vi "Destroy.vi"(0 "reference in":refnum<class "LcPictureBox.lvclass">, 5 "Error In":errorcluster) -> (14 "reference out":refnum<class "LcPictureBox.lvclass">, 19 "Error Out":errorcluster)   [LabVIEW 2020, in "LcPictureBox.lvclass"]
uses:
  LcPictureBox.lvclass
  System.Drawing
  System.Windows.Forms
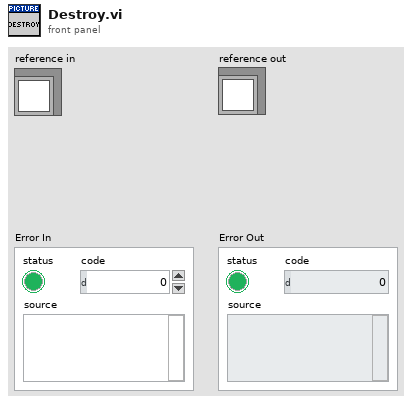
[diagram p1: front panel]
types:
  T1 = typedef "LcPictureBox.lvclass/ObjectAttributes.ctl" = cluster{"PictureBox":refnum<k24>, "ImageSize":cluster{"Width":i32, "Height":i32}, "PenMemory":map{cluster{"Alpha(100%)":dbl, "Color(Black)":u32, "Pen(Width=1, Solid)":T2}, refnum<k24>}, "GraphicsRef":refnum<k24>, "BrushMemory":map{cluster{"Alpha(100%)":dbl, "Color(Black)":u32}, refnum<k24>}, "Images":refnum<k24>[], "ImageIndex":i32, "BgColor(None)":u32, "LoadedImages":map{string, cluster{"ImageOut":refnum<k24>, "ImageSize":cluster{"Width":i32, "Height":i32}}}, "ColorsMemory":map{cluster{"Alpha(100%)":dbl, "Color(Black)":u32}, refnum<k24>}, "CacheSize":i32, "PictureBoxActiveXReference":refnum<vi>, "Scale":dbl, "Offset":cluster{"x":sgl, "y":sgl}, "zoom_center":cluster{"X":i32, "Y":i32}, "ImagesCreated":refnum<k24>[], "CustomCursorImages":map{u16, refnum<k24>}}
  T2 = typedef "LcPictureBox.lvclass/Pen.ctl" = cluster{"Width":u16, "Style":enum32{"Solid", "Dash", "Dot", "DashDot", "DashDotDot"}}
  T3 = map{cluster{"Alpha(100%)":dbl, "Color(Black)":u32}, refnum<k24>}
  T4 = map{cluster{"Alpha(100%)":dbl, "Color(Black)":u32, "Pen(Width=1, Solid)":T2}, refnum<k24>}
  T5 = map{string, cluster{"ImageOut":refnum<k24>, "ImageSize":cluster{"Width":i32, "Height":i32}}}
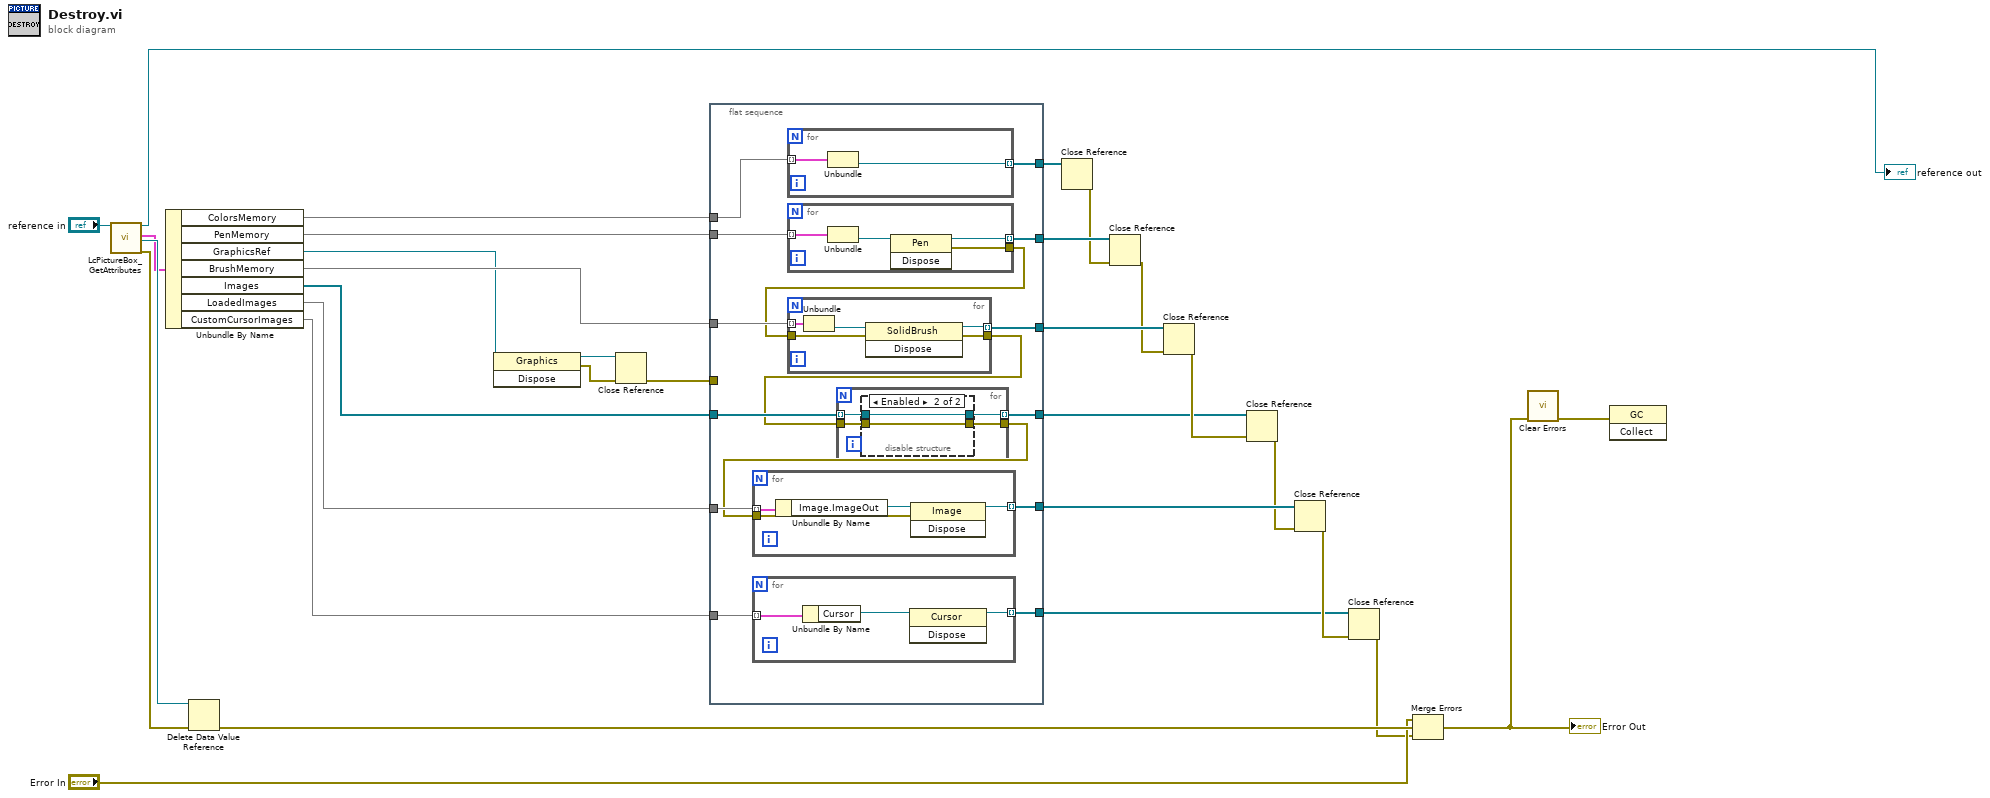
[diagram p0: block diagram]
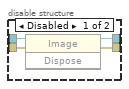
[diagram p2: hidden frame]
diagram:
  n1 = call "LcPictureBox_GetAttributes.vi"("reference in"="reference in") -> ("reference out"=→"reference out":refnum<class "LcPictureBox.lvclass">, "Data"=w27:T1, "DataRef"=w28:refnum<data-value>, "error out"=w29:errorcluster)  [unwired: 15 in]
  n2 = Unbundle By Name(w27) -> ("ColorsMemory"=w20:T3, "PenMemory"=w24:T4, "GraphicsRef"=w1:refnum<k24>, "BrushMemory"=w23:T3, "Images"=w22:refnum<k24>[], "LoadedImages"=w21:T5, "CustomCursorImages"=w5:map{u16, refnum<k24>})
  n3 = Delete Data Value Reference(data value reference=w28, error in=w29) -> (error out=w26:errorcluster)  [unwired: 1 out]
  n4 = invoke class="Graphics" method="Dispose"(reference=w1) -> (reference out=w19:refnum<k24>, error out=w18:errorcluster)  [unwired: 2 in, 1 out]
  n5 = Close Reference(reference=w19, error in (no error)=w18) -> (error out=w8:errorcluster)
  n6 = flat-sequence {
    tunnel: w24 -> [w46]
    tunnel: [w45] -> w17
    tunnel: w23 -> [w44]
    tunnel: [w43] -> w16
    tunnel: w22 -> [w42]
    tunnel: [w41] -> w13
    tunnel: w21 -> [w40]
    tunnel: [w39] -> w12
    tunnel: w20 -> [w35]
    tunnel: [w34] -> w10
    tunnel: w8 -> [_]
    tunnel: w5 -> [w33]
    tunnel: [w32] -> w2
    frame #0 {
      n7 = for {
        tunnel: w33 -> [w48] mode=indexing
        tunnel: [w49] -> w32 mode=indexing
        n8 = Unbundle By Name(w48) -> ("Cursor"=w47:refnum<k24>)
        n9 = invoke class="Cursor" method="Dispose"(reference=w47) -> (reference out=w49:refnum<k24>)  [unwired: 2 in, 2 out]
      }
      n10 = for {
        tunnel: w35 -> [w51] mode=indexing
        tunnel: [w50] -> w34 mode=indexing
        n11 = Unbundle(w51) -> ("ColorRef"=w50:refnum<k24>)  [unwired: 1 out]
      }
      n12 = for {
        tunnel: w46 -> [w74] mode=indexing
        tunnel: [w72] -> w45 mode=indexing
        tunnel: [w71] -> w38
        n13 = Unbundle(w74) -> ("PenRef"=w73:refnum<k24>)  [unwired: 1 out]
        n14 = invoke class="Pen" method="Dispose"(reference=w73) -> (reference out=w72:refnum<k24>, error out=w71:errorcluster)  [unwired: 2 in, 1 out]
      }
      n15 = for {
        tunnel: w44 -> [w70] mode=indexing
        tunnel: [w68] -> w43 mode=indexing
        tunnel: w38 -> [w67]
        tunnel: [w66] -> w37
        n16 = Unbundle(w70) -> ("PenRef"=w69:refnum<k24>)  [unwired: 1 out]
        n17 = invoke class="SolidBrush" method="Dispose"(reference=w69, error in=w67) -> (reference out=w68:refnum<k24>, error out=w66:errorcluster)  [unwired: 1 in, 1 out]
      }
      n18 = for {
        tunnel: w42 -> [w59] mode=indexing
        tunnel: [w58] -> w41 mode=indexing
        tunnel: w37 -> [w57]
        tunnel: [w56] -> w36
        n19 = disable-structure shown="Enabled" {
          disable-tunnel: w59 -> [w63 w65]
          disable-tunnel: [w62 w65] -> w58
          disable-tunnel: w57 -> [w61 w64]
          disable-tunnel: [w60 w64] -> w56
          frame Disabled {
            n20 = invoke class="Image" method="Dispose"(reference=w63, error in=w61) -> (reference out=w62:refnum<k24>, error out=w60:errorcluster)  [unwired: 1 in, 1 out]
          }
          frame Enabled {
          }
        }
      }
      n21 = for {
        tunnel: w40 -> [w54] mode=indexing
        tunnel: [w55] -> w39 mode=indexing
        tunnel: w36 -> [w52]
        n22 = Unbundle By Name(w54) -> ("Image.ImageOut"=w53:refnum<k24>)
        n23 = invoke class="Image" method="Dispose"(reference=w53, error in=w52) -> (reference out=w55:refnum<k24>)  [unwired: 1 in, 2 out]
      }
    }
  }
  n24 = Close Reference(reference=w10) -> (error out=w9:errorcluster)  [unwired: 1 in]
  n25 = Close Reference(reference=w17, error in (no error)=w9) -> (error out=w15:errorcluster)
  n26 = Close Reference(reference=w16, error in (no error)=w15) -> (error out=w14:errorcluster)
  n27 = Close Reference(reference=w13, error in (no error)=w14) -> (error out=w11:errorcluster)
  n28 = Close Reference(reference=w12, error in (no error)=w11) -> (error out=w4:errorcluster)
  n29 = Close Reference(reference=w2, error in (no error)=w4) -> (error out=w3:errorcluster)
  n30 = Merge Errors("Error In", w26, w3) -> (w7:errorcluster)
  "Error Out" <- w7
  n31 = call <vilib>:"Clear Errors.vi"("error in (no error)"=w7) -> ("error out"=w6:errorcluster)  [unwired: 5 in, 1 out]
  n32 = invoke class="GC" method="Collect"(error in=w6) -> ()  [unwired: 2 in, 3 out]
